vi "Read Timing Source Properties.vi"(8 "error in (no error)":errorcluster, 11 "TimingSource in":refnum<class "TimingSource.lvclass">) -> (0 "error out":errorcluster, 2 "Timing Source":T1, 3 "TimingSource out":refnum<class "TimingSource.lvclass">)   [LabVIEW 2015, in "TimingSource.lvclass"]
uses:
  TimingSource.lvclass
  Custom Device Type Defs/Timing Source Properties.ctl
  XML Controls/Source Distribution for TimingSource.ctl
  XML Controls/Target.ctl
  XML Controls/Path Cluster.ctl
  TimingSource.lvclass/TimingSource.ctl
  Configuration Tool.lvlib
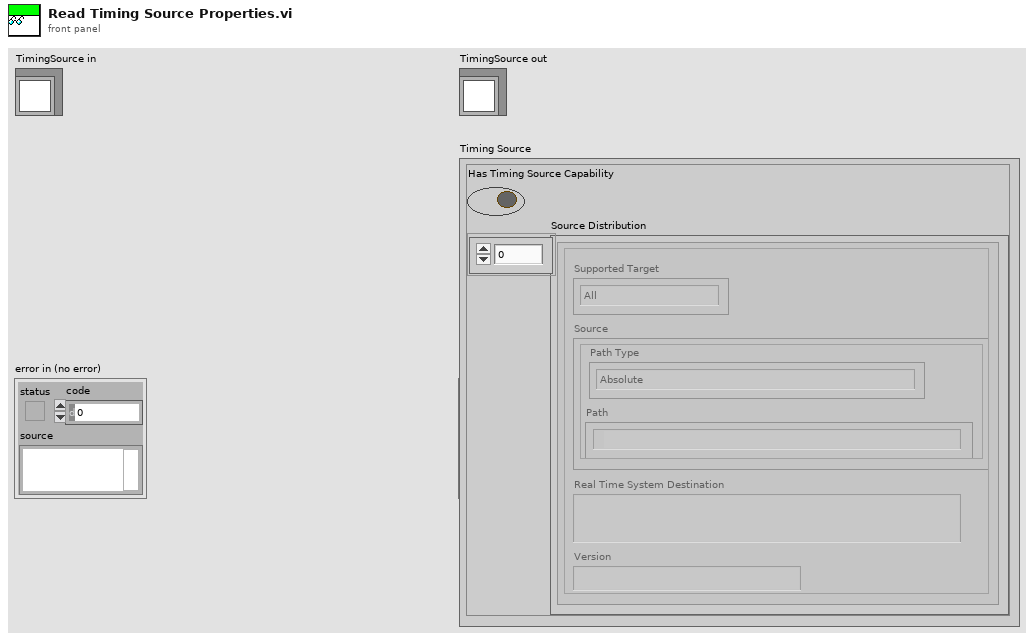
[diagram p1: front panel]
types:
  T1 = typedef "Timing Source Properties.ctl" = cluster{"Has Timing Source Capability":bool, "Source Distribution":T2}
  T2 = typedef "Configuration Tool.lvlib/Source Distribution for TimingSource.ctl" = cluster{"Supported Target":T3, "Source":T4, "Real Time System Destination":string, "Version":string}[]
  T3 = typedef "Configuration Tool.lvlib/Target.ctl" = enum16{"All", "Pharlap", "VxWorks", "Windows", "Linux_32_ARM", "Linux_x64", "PharlapWindows", "PharlapVxWorks", "VxWorksWindows"}
  T4 = typedef "Configuration Tool.lvlib/Path Cluster.ctl" = cluster{"Path":path, "Path Type":enum16{"Absolute", "To Base", "To Common Doc Dir", "To Application Data Dir"}}
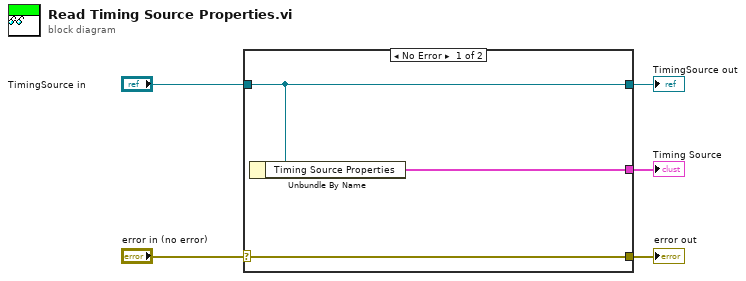
[diagram p0: block diagram]
diagram:
  n1 = case shown="No Error" "error in (no error)" {
    selector: "error in (no error)" -> [w8 w9]
    tunnel: [w8 w9] -> w4
    tunnel: [w7 w10] -> w2
    tunnel: "TimingSource in" -> [w7 w10]
    tunnel: [w6 _] -> w1
    frame No Error {
      n2 = Unbundle By Name(w7) -> ("Timing Source Properties"=w6:T1)
    }
    frame Error {
    }
  }
  "error out" <- w4
  "TimingSource out" <- w2
  "Timing Source" <- w1
